vi "CMD_08T_SetSetpoint.vi"(9 "Setpoint, K":dbl=295.0 min=195.0 max=400.0, 11 "VISA resource name":refnum<visa-resource-name>) -> (3 "VISA resource name out":refnum<visa-resource-name>)   [LabVIEW 2013]
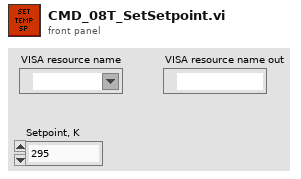
[diagram p1: front panel]
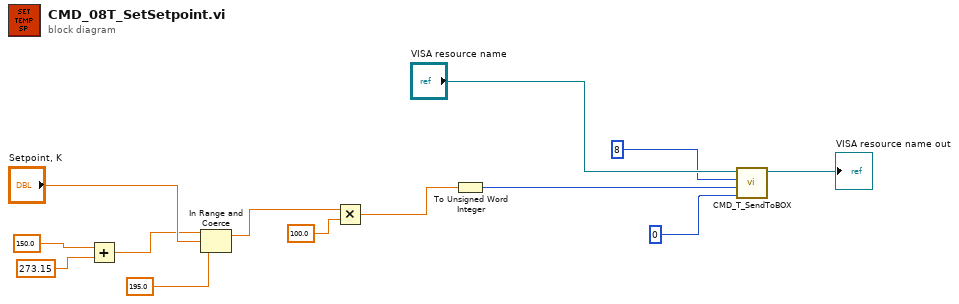
[diagram p0: block diagram]
diagram:
  n1 = Add(x=150.0, y=273.15) -> (x+y=w1:dbl)
  n2 = In Range and Coerce(upper limit=w1, x="Setpoint, K", lower limit=195.0) -> (coerced(x)=w4:dbl)  [unwired: 1 out]
  n3 = Multiply(x=w4, y=100.0) -> (x*y=w8:dbl)
  n4 = To Unsigned Word Integer(number=w8) -> (unsigned 16bit integer=w10:u16)
  n5 = call "CMD_T_SendToBOX.vi"("arg2"=i16 0, "arg1"=w10, "CMD"=i8 8, "VISA resource name"="VISA resource name") -> ("VISA resource name out"=→"VISA resource name out":refnum<visa-resource-name>)  [unwired: 7 in]
